vi "gentec-M-Link.Start Data Flow.vi"(0 "VISA resource In":refnum<visa-resource-name>, 5 "error in (no error)":errorcluster) -> (14 "VISA resource Out":refnum<visa-resource-name>, 19 "error out":errorcluster)   [LabVIEW 2014, in "gentec-M-Link - Driver.lvlib"]
doc: "Data to write: str1\n\nStarts the data flow. Data is sent at the pulse rate for Energy, at the chop rate for Radiometers, and at 10Hz for Power. Data is sent as certain hexadecimal data string."
uses:
  gentec-M-Link - Driver.lvlib
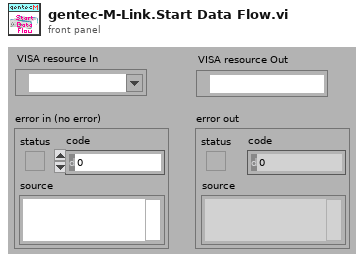
[diagram p1: front panel]
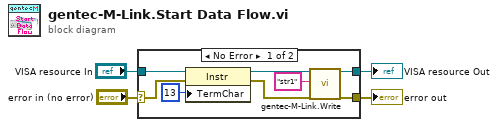
[diagram p0: block diagram]
diagram:
  n1 = case shown="No Error" "error in (no error)" {
    selector: "error in (no error)" -> [w7 w14]
    tunnel: [w10 w14] -> w3
    tunnel: "VISA resource In" -> [w9 w13]
    tunnel: [w11 w13] -> w1
    frame No Error {
      n2 = property class="Instr"(reference=w9, error in=w7, "TermChar"=u8 13 ("Message Based Settings:Termination Character")) -> (reference out=w8:refnum<visa-resource-name>, error out=w6:errorcluster)
      n3 = call "gentec-M-Link.Write.vi"("VISA resource (In)"=w8, "Data To Write"="str1", "error in (no error)"=w6) -> ("VISA resource (Out)"=w11:refnum<visa-resource-name>, "error out"=w10:errorcluster)  [unwired: 14 in, 1 out]
    }
    frame Error {
    }
  }
  "error out" <- w3
  "VISA resource Out" <- w1
